vi "Inspect TBM.vi"(7 "Console Log in":refnum<class "Console Log.lvclass">, 8 "error in":errorcluster, 10 "Module Data In":T1={"TBM-TBM"={"Fiducial Image"={"Image Position"=refnum, "Image Reference"=refnum, "Field of View"={"x(mm)"=0.0, "y(mm)"=0.0}}, "Fiducials"=[]}, "TBM-HDI"={"Fiducial Image"={"Image Position"=refnum, "Image Reference"=refnum, "Field of View"={"x(mm)"=0.0, "y(mm)"=0.0}}, "Fiducials"=[]}, "Address Pads"={"Fiducial Image"={"Image Position"=refnum, "Image Reference"=refnum, "Field of View"={"x(mm)"=0.0, "y(mm)"=0.0}}, "Fiducials"=[]}, "HDI Bond Pad References"=[], "BBM Bond Pad References"=[], "HV-HDI"={"Fiducial Image"={"Image Position"=refnum, "Image Reference"=refnum, "Field of View"={"x(mm)"=0.0, "y(mm)"=0.0}}, "Selected Fiducial"={"Fiducial Image Coordinate"=refnum, "Fiducial Source"=enum."Pattern Recognition"}, "fiducial name"=""}, "HV-BBM"={"Fiducial Image"={"Image Position"=refnum, "Image Reference"=refnum, "Field of View"={"x(mm)"=0.0, "y(mm)"=0.0}}, "Selected Fiducial"={"Fiducial Image Coordinate"=refnum, "Fiducial Source"=enum."Pattern Recognition"}, "fiducial name"=""}, "Chuck"=0, "Slot"=0, "Potting Selection"={"HDI Bond Pads"=[TRUE, TRUE, TRUE, TRUE, TRUE, TRUE, TRUE, TRUE, TRUE, TRUE, TRUE, TRUE, TRUE, TRUE, TRUE, TRUE], "BBM Bond Pads"=[TRUE, TRUE, TRUE, TRUE, TRUE, TRUE, TRUE, TRUE, TRUE, TRUE, TRUE, TRUE, TRUE, TRUE, TRUE, TRUE], "TBM Inner"={"Top"=TRUE, "Left"=TRUE, "Bottom"=TRUE, "Right"=TRUE}, "TBM Outer"={"Top"=TRUE, "Left"=TRUE, "Bottom"=TRUE, "Right"=TRUE}, "Address Pads"={"Top"=TRUE, "Bottom"=TRUE}, "High Voltage"={"HDI"=TRUE, "BBM"=TRUE}}}, 11 "Potting Procedure in":refnum<class "Potting Procedure.lvclass">) -> (0 "error out":errorcluster, 2 "Module Data Out":T1={"TBM-TBM"={"Fiducial Image"={"Image Position"=refnum, "Image Reference"=refnum, "Field of View"={"x(mm)"=0.0, "y(mm)"=0.0}}, "Fiducials"=[]}, "TBM-HDI"={"Fiducial Image"={"Image Position"=refnum, "Image Reference"=refnum, "Field of View"={"x(mm)"=0.0, "y(mm)"=0.0}}, "Fiducials"=[]}, "Address Pads"={"Fiducial Image"={"Image Position"=refnum, "Image Reference"=refnum, "Field of View"={"x(mm)"=0.0, "y(mm)"=0.0}}, "Fiducials"=[]}, "HDI Bond Pad References"=[], "BBM Bond Pad References"=[], "HV-HDI"={"Fiducial Image"={"Image Position"=refnum, "Image Reference"=refnum, "Field of View"={"x(mm)"=0.0, "y(mm)"=0.0}}, "Selected Fiducial"={"Fiducial Image Coordinate"=refnum, "Fiducial Source"=enum."Pattern Recognition"}, "fiducial name"=""}, "HV-BBM"={"Fiducial Image"={"Image Position"=refnum, "Image Reference"=refnum, "Field of View"={"x(mm)"=0.0, "y(mm)"=0.0}}, "Selected Fiducial"={"Fiducial Image Coordinate"=refnum, "Fiducial Source"=enum."Pattern Recognition"}, "fiducial name"=""}, "Chuck"=0, "Slot"=0, "Potting Selection"={"HDI Bond Pads"=[TRUE, TRUE, TRUE, TRUE, TRUE, TRUE, TRUE, TRUE, TRUE, TRUE, TRUE, TRUE, TRUE, TRUE, TRUE, TRUE], "BBM Bond Pads"=[TRUE, TRUE, TRUE, TRUE, TRUE, TRUE, TRUE, TRUE, TRUE, TRUE, TRUE, TRUE, TRUE, TRUE, TRUE, TRUE], "TBM Inner"={"Top"=TRUE, "Left"=TRUE, "Bottom"=TRUE, "Right"=TRUE}, "TBM Outer"={"Top"=TRUE, "Left"=TRUE, "Bottom"=TRUE, "Right"=TRUE}, "Address Pads"={"Top"=TRUE, "Bottom"=TRUE}, "High Voltage"={"HDI"=TRUE, "BBM"=TRUE}}}, 3 "Potting Procedure out":refnum<class "Potting Procedure.lvclass">, 5 "Console Log out":refnum<class "Console Log.lvclass">)   [LabVIEW 2017, in "Potting Procedure.lvclass"]
uses:
  Potting Procedure.lvclass
  Shared Components/CameraTool Class/CameraTool Class.lvclass
  Shared Components/Vec3d Class/Vec3d Class.lvclass
  Shared Components/Utils/Type Definitions/Fiducial with Source.ctl
  Shared Components/WorkTable Class/WorkTable Class.lvclass
  Shared Components/Gantry Class/Gantry Class.lvclass
  Application Utilities/Console Log/Console Log.lvclass
  Shared Components/Config Manager Class/Config Manager Class.lvclass
  Shared Components/Config Manager Class/Read Geometry Definition 3D.vi
  Shared Components/Config Manager Class/Type Definitions/Part Type.ctl
  Shared Components/CameraTool Class/Take Area Image.vi
  Shared Components/CameraTool Class/Take Outline Image.vi
  Shared Components/Config Manager Class/Read Geometry Definition Double.vi
  <vilib>/vision/Image Controls.llb/IMAQ Image.ctl
  Shared Components/Utils/Type Definitions/Physical Image.ctl
  Shared Components/Utils/Type Definitions/Multi-Fiducial Image.ctl
  Shared Components/Utils/Type Definitions/Fiducial Image.ctl
  Type Definitions/Inspect Modules - Module.ctl
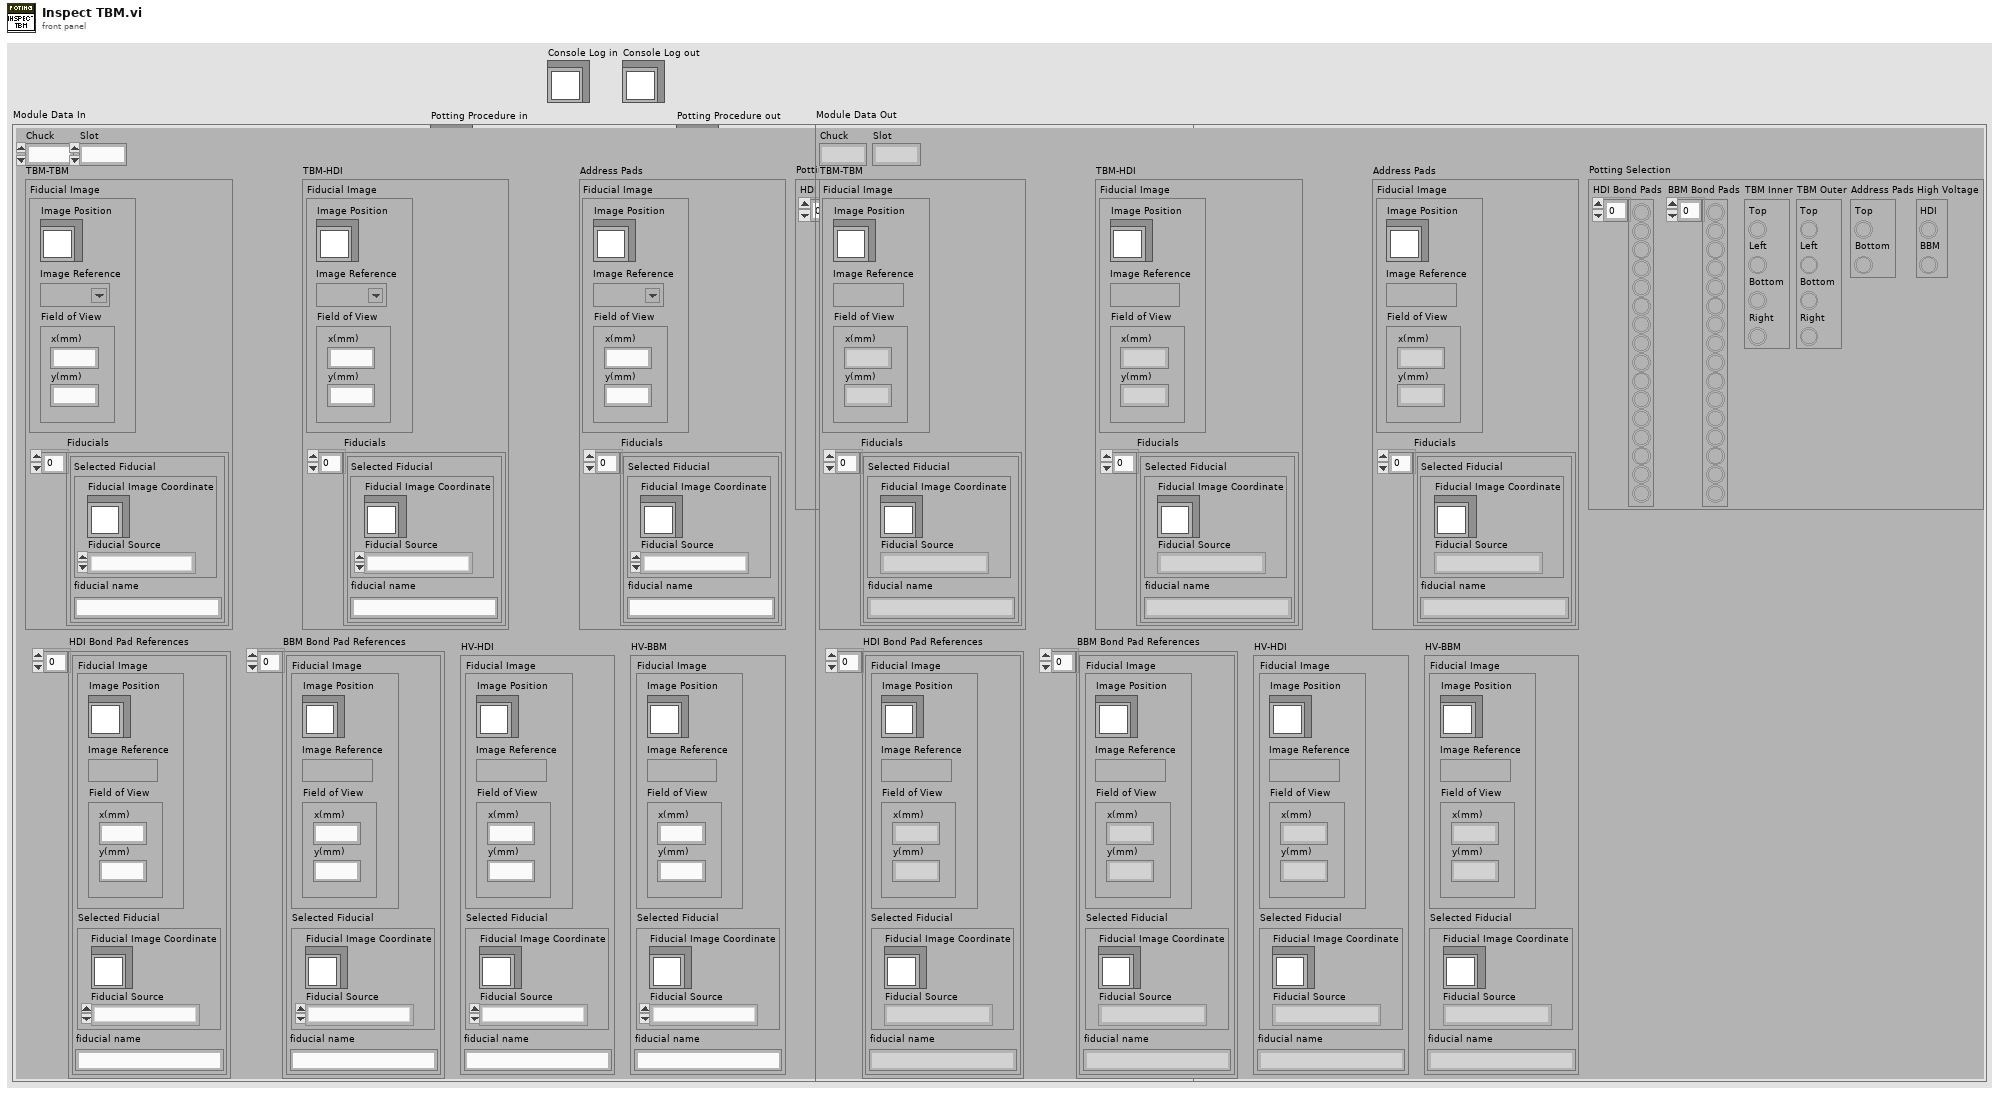
[diagram p1: front panel]
types:
  T1 = typedef "Inspect Modules - Module.ctl" = cluster{"TBM-TBM":T2, "TBM-HDI":T2, "Address Pads":T2, "HDI Bond Pad References":T6[], "BBM Bond Pad References":T6[], "HV-HDI":T6, "HV-BBM":T6, "Chuck":i32, "Slot":i32, "Potting Selection":cluster{"HDI Bond Pads":bool[], "BBM Bond Pads":bool[], "TBM Inner":cluster{"Top":bool, "Left":bool, "Bottom":bool, "Right":bool}, "TBM Outer":cluster{"Top":bool, "Left":bool, "Bottom":bool, "Right":bool}, "Address Pads":cluster{"Top":bool, "Bottom":bool}, "High Voltage":cluster{"HDI":bool, "BBM":bool}}}
  T2 = typedef "Multi-Fiducial Image.ctl" = cluster{"Fiducial Image":T3, "Fiducials":cluster{"Selected Fiducial":T5, "fiducial name":string}[]}
  T3 = typedef "Physical Image.ctl" = cluster{"Image Position":refnum<class "Vec3d Class.lvclass">, "Image Reference":T4, "Field of View":cluster{"x(mm)":dbl, "y(mm)":dbl}}
  T4 = typedef "IMAQ Image.ctl" = refnum<image>
  T5 = typedef "Fiducial with Source.ctl" = cluster{"Fiducial Image Coordinate":refnum<class "Vec3d Class.lvclass">, "Fiducial Source":enum16{"Pattern Recognition", "User", "Error", "Default"}}
  T6 = typedef "Fiducial Image.ctl" = cluster{"Fiducial Image":T3, "Selected Fiducial":T5, "fiducial name":string}
  T7 = enum16{"Pattern Recognition", "User", "Error", "Default"}
  T8 = cluster{"Selected Fiducial":T5, "fiducial name":string}
  T9 = typedef "Part Type.ctl" = enum16{"BBM", "HDI", "BARE HDI", "GLUERESERVOIR", "STAMP_1", "STAMP_2", "STAMP_3", "STAMP_4", "STAMP_5", "WEIGHT_1", "WEIGHT_2", "WEIGHT_3", "WEIGHT_4", "WEIGHT_5", "WEIGHT_6", "WEIGHT_7", "WEIGHT_8", "PICKER_TOOL", "GRABER_TOOL"}
  T10 = typedef "Worktable_Module Slot.ctl" = cluster{"Slot State":enum16{"Empty", "Bare HDI", "Unglued", "Stamped", "PartOnTop", "Weighted", "Unpotted", "Potted"}, "BBM Type":enum16{"None", "BBM", "GlassSlide"}, "HDI Type":enum16{"None", "HDI", "Polyimide"}, "Vacuum Channel":u8, "Location/Orientation BBM":T11, "Location/Orientation HDI":T11, "S/N":string}
  T11 = typedef "Position_Orientation.ctl" = cluster{"Center":refnum<class "Vec3d Class.lvclass">, "Orientation":refnum<class "Orient3d Class.lvclass">}
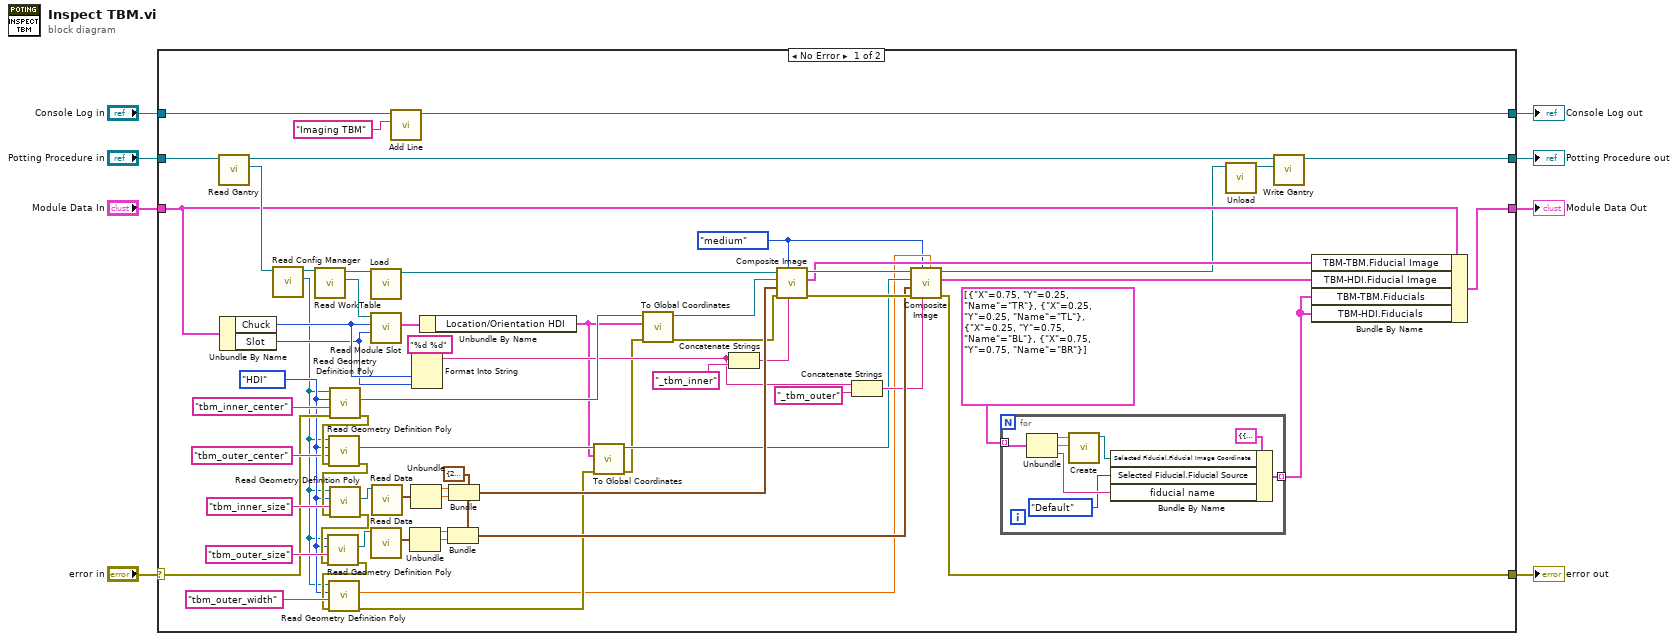
[diagram p0: block diagram]
diagram:
  n1 = case shown="No Error" "error in" {
    selector: "error in" -> [w20 w84]
    tunnel: [w45 w84] -> w7
    tunnel: [w29 w83] -> w5
    tunnel: "Potting Procedure in" -> [w72 w83]
    tunnel: "Module Data In" -> [w36 w82]
    tunnel: [w31 w82] -> w1
    tunnel: "Console Log in" -> [w26 w81]
    tunnel: [w25 w81] -> w3
    frame No Error {
      w9 = enum16{"perfect", "high", "medium", "low"}."medium" ("Quality")
      w13 = Part_Type."HDI" ("Part Type")
      w54 = cluster{"Size-X(mm)":dbl, "Size-Y(mm)":dbl} {"Size-X(mm)"=20.0, "Size-Y(mm)"=20.0} ("Field of View")
      n2 = call-dynamic "Read Gantry.vi"("Potting Procedure in"=w72) -> ("Gantry"=w70:refnum<class "Gantry Class.lvclass">, "Potting Procedure out"=w28:refnum<class "Potting Procedure.lvclass">)  [unwired: 8 in, 1 out]
      n3 = Unbundle By Name(w36) -> ("Chuck"=w38:i32, "Slot"=w37:i32)
      n4 = call-dynamic "Read Config Manager.vi"("Gantry in"=w70) -> ("Config Manager"=w12:refnum<class "Config Manager Class.lvclass">, "Gantry out"=w52:refnum<class "Gantry Class.lvclass">)  [unwired: 8 in, 1 out]
      n5 = call-dynamic "Read WorkTable.vi"("Gantry Class in"=w52) -> ("Worktable"=w50:refnum<class "FlexWorktable.lvclass">, "Gantry Class out"=w51:refnum<class "Gantry Class.lvclass">)  [unwired: 8 in, 1 out]
      n6 = call-poly "Read Geometry Definition Poly.vi"("error in"=w20, "Feature"="tbm_inner_center", "Part Type"=w13, "Config Manager in"=w12) -> ("error out"=w22:errorcluster, "Feature Coordinates"=w48:refnum<class "Vec3d Class.lvclass">)  [unwired: 5 in, 1 out]
      n7 = call-poly "Read Geometry Definition Poly.vi"("error in"=w22, "Feature"="tbm_outer_center", "Part Type"=w13, "Config Manager in"=w12) -> ("error out"=w23:errorcluster, "Feature Coordinates"=w19:refnum<class "Vec3d Class.lvclass">)  [unwired: 5 in, 1 out]
      n8 = call-poly "Read Geometry Definition Poly.vi"("error in"=w23, "Feature"="tbm_inner_size", "Part Type"=w13, "Config Manager in"=w12) -> ("error out"=w66:errorcluster, "Feature Coordinates"=w63:refnum<class "Vec3d Class.lvclass">)  [unwired: 5 in, 1 out]
      n9 = call-poly "Read Geometry Definition Poly.vi"("error in"=w66, "Feature"="tbm_outer_size", "Part Type"=w13, "Config Manager in"=w12) -> ("error out"=w14:errorcluster, "Feature Coordinates"=w55:refnum<class "Vec3d Class.lvclass">)  [unwired: 5 in, 1 out]
      n10 = call-poly "Read Geometry Definition Poly.vi"("error in"=w14, "Feature"="tbm_outer_width", "Part Type"=w13, "Config Manager in"=w12) -> ("error out"=w11:errorcluster, "Geometry Definition"=w10:dbl)  [unwired: 5 in, 1 out]
      n11 = call "Load.vi"("Gantry In"=w51) -> ("CameraTool out"=w71:refnum<class "CameraTool Class.lvclass">)  [unwired: 9 in, 1 out]
      n12 = call-dynamic "Read Module Slot.vi"("slot"=w37, "chuck"=w38, "WorkTable in"=w50) -> ("Module Slot"=w49:T10)  [unwired: 6 in, 2 out]
      n13 = call-dynamic "Read Data.vi"("Vec3d Class in"=w55) -> ("Data"=w58:cluster{"X":dbl, "Y":dbl, "Z":dbl})  [unwired: 8 in, 2 out]
      n14 = call-dynamic "Read Data.vi"("Vec3d Class in"=w63) -> ("Data"=w62:cluster{"X":dbl, "Y":dbl, "Z":dbl})  [unwired: 8 in, 2 out]
      n15 = call "Add Line.vi"("String"="Imaging TBM", "Console Log in"=w26) -> ("Console Log out"=w25:refnum<class "Console Log.lvclass">)  [unwired: 8 in, 1 out]
      n16 = Unbundle(w58) -> ("X"=w57:dbl, "Y"=w56:dbl)  [unwired: 1 out]
      n17 = Unbundle(w62) -> ("X"=w61:dbl, "Y"=w60:dbl)  [unwired: 1 out]
      n18 = Format Into String(format string="%d %d", w38, w37) -> (resulting string=w41:string)  [unwired: 2 in, 1 out]
      n19 = Unbundle By Name(w49) -> ("Location/Orientation HDI"=w17:T11)
      n20 = Bundle(cluster=w54, "Size-X(mm)"=w57, "Size-Y(mm)"=w56) -> (w53:cluster{"Size-X(mm)":dbl, "Size-Y(mm)":dbl})
      n21 = Bundle(cluster=w54, "Size-X(mm)"=w61, "Size-Y(mm)"=w60) -> (w59:cluster{"Size-X(mm)":dbl, "Size-Y(mm)":dbl})
      n22 = call "To Global Coordinates.vi"("error in"=w11, "Center/Orientation"=w17, "Local Coordinates"=w19) -> ("error out"=w16:errorcluster, "Global Coordinates"=w18:refnum<class "Vec3d Class.lvclass">)  [unwired: 7 in]
      n23 = call "To Global Coordinates.vi"("error in"=w16, "Center/Orientation"=w17, "Local Coordinates"=w48) -> ("error out"=w47:errorcluster, "Global Coordinates"=w46:refnum<class "Vec3d Class.lvclass">)  [unwired: 7 in]
      n24 = Concatenate Strings(w41, "_tbm_inner" ("string")) -> (w40:string)
      n25 = call-poly "Composite Image.vi"("Image Name"=w40, "Quality"=w9, "error in"=w47, "Field of View"=w59, "Image Center"=w46, "CameraTool in"=w71) -> ("error out"=w64:errorcluster, "Physical Image"=w35:T3, "CameraTool out"=w65:refnum<class "CameraTool Class.lvclass">)  [unwired: 3 in]
      n26 = Concatenate Strings(w41, "_tbm_outer" ("string")) -> (w39:string)
      n27 = call-poly "Composite Image.vi"("Outline Width"=w10, "Image Name"=w39, "Quality"=w9, "error in"=w64, "Field of View"=w53, "Image Center"=w18, "CameraTool in"=w65) -> ("error out"=w45:errorcluster, "Physical Image"=w34:T3, "CameraTool out"=w30:refnum<class "CameraTool Class.lvclass">)  [unwired: 2 in]
      n28 = for {
        tunnel: cluster{"X":dbl, "Y":dbl, "Name":string}[] [{"X"=0.75, "Y"=0.25, "Name"="TR"}, {"X"=0.25, "Y"=0.25, "Name"="TL"}, {"X"=0.25, "Y"=0.75, "Name"="BL"}, {"X"=0.75, "Y"=0.75, "Name"="BR"}] -> [w79] mode=indexing
        tunnel: [w73] -> w32 mode=indexing
        n29 = Unbundle(w79) -> ("X"=w77:dbl, "Y"=w78:dbl, "Name"=w75:string)
        n30 = call "Create.vi"("Y"=w78, "X"=w77) -> ("Vec3d Class out"=w76:refnum<class "Vec3d Class.lvclass">)  [unwired: 8 in, 1 out]
        n31 = Bundle By Name(cluster=T8 {"Selected Fiducial"={"Fiducial Image Coordinate"=refnum, "Fiducial Source"=enum."Pattern Recognition"}, "fiducial name"=""} ("Fiducial"), "Selected Fiducial.Fiducial Image Coordinate"=w76, "Selected Fiducial.Fiducial Source"=T7."Default", "fiducial name"=w75) -> (w73:T8)
      }
      n32 = call "Unload.vi"("CameraTool in"=w30) -> ("Gantry out"=w27:refnum<class "Gantry Class.lvclass">)  [unwired: 9 in, 1 out]
      n33 = call-dynamic "Write Gantry.vi"("Gantry"=w27, "Potting Procedure in"=w28) -> ("Potting Procedure out"=w29:refnum<class "Potting Procedure.lvclass">)  [unwired: 8 in, 1 out]
      n34 = Bundle By Name(cluster=w36, "TBM-TBM.Fiducial Image"=w35, "TBM-HDI.Fiducial Image"=w34, "TBM-TBM.Fiducials"=w32, "TBM-HDI.Fiducials"=w32) -> (w31:T1)
    }
    frame Error {
    }
  }
  "error out" <- w7
  "Potting Procedure out" <- w5
  "Console Log out" <- w3
  "Module Data Out" <- w1
